vi "Set Animations.vi"(8 "Error In":errorcluster, 10 "Animations":refnum<class "Animation.lvclass">[](array[class]), 11 "Display Manager In":refnum<class "Display Manager.lvclass">) -> (0 "Error Out":errorcluster, 3 "Display Manager Out":refnum<class "Display Manager.lvclass">)   [LabVIEW 2021, in "Display Manager.lvclass"]
uses:
  Display Manager.lvclass
  Display Manager.lvclass/Display Manager.ctl
  Animation/Animation.lvclass
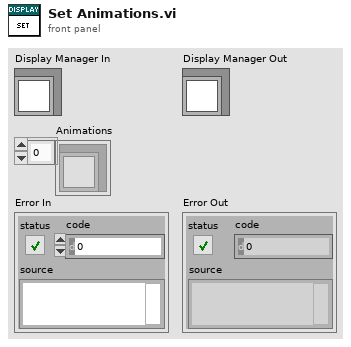
[diagram p1: front panel]
types:
  T1 = typedef "Display Manager.lvclass/Data.ctl" = cluster{"Size":T2, "Display Elements":refnum<class "Display Element.lvclass">[], "Frame":u32[][], "Animations":refnum<class "Animation.lvclass">[]}
  T2 = typedef "Display Utilities.lvlib/2D Dimensions.ctl" = cluster{"Width":i32, "Height":i32}
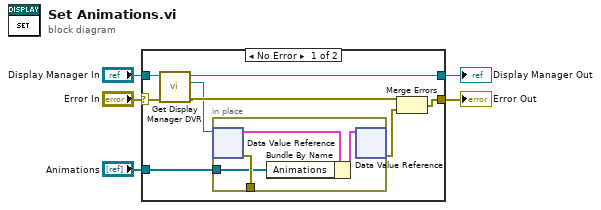
[diagram p0: block diagram]
diagram:
  n1 = case shown="No Error" "Error In" {
    selector: "Error In" -> [w9 w18]
    tunnel: [w12 w18] -> w2
    tunnel: [w8 w19] -> w5
    tunnel: "Display Manager In" -> [w10 w19]
    tunnel: "Animations" -> [w11 _]
    frame No Error {
      n2 = call "Get Display Manager DVR.vi"("Error In"=w9, "Display Manager In"=w10) -> ("Error Out"=w7:errorcluster, "DVR"=w6:refnum<data-value>, "Display Manager Out"=w8:refnum<class "Display Manager.lvclass">)  [unwired: 7 in]
      n3 = in-place {
        in-place-border: [w17] -> _
        in-place-border: w11 -> [w14]
        n4 = in-place-dvr #1(w6) -> (w16:T1, w17:errorcluster)
        n5 = Bundle By Name(cluster=w16, "Animations"=w14) -> (w15:T1)
        n6 = in-place-dvr #1(w15) -> (w13:errorcluster)  [unwired: 1 out]
      }
      n7 = Merge Errors(w7, w13) -> (w12:errorcluster)
    }
    frame Error {
    }
  }
  "Display Manager Out" <- w5
  "Error Out" <- w2
